vi "RSZVB Get Source Power Calibration Port State.vi"(8 "error in (no error)":errorcluster {"code" format="%.0x"}, 9 "Port Number (1)":i32=1, 10 "Channel (1)":i32=1, 11 "VISA session":refnum<visa-resource-name>) -> (0 "error out":errorcluster {"code" format="%.0x"}, 2 "Port State":bool, 3 "dup VISA session":refnum<visa-resource-name>)   [LabVIEW 2011]
doc: "This VI returns the state of the source power calibration for channel <Ch> and for port number <Pt>. \n\nNotes:\n\n(1) The command is disabled unless a source power calibration for the analyzer port has been performed (rszvb_InitiateSourcePowerCalibration). \n\n(2) To enable or disable a source power calibration for an external generator use SOURce<Ch>:POWer<Pt>:CORRection:GENerator[:STATe].\n\nRemote-control command(s):\nSOURce<Ch>:POWer<Pt>:CORRection[:STATe]?"
uses:
  _utility/RSZVB Global Data.vi
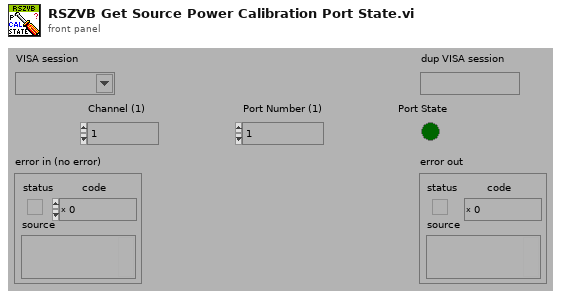
[diagram p1: front panel]
types:
  T1 = cluster{"Error Checking (T: On)":bool, "Installed Options":string[], "Data Valid?":bool, "Ports":i32, "Model":string[], "Option Checking (T: On)":bool}[]
  T2 = cluster{"Error Checking (T: On)":bool, "Installed Options":string[], "Data Valid?":bool, "Ports":i32, "Model":string[], "Option Checking (T: On)":bool}
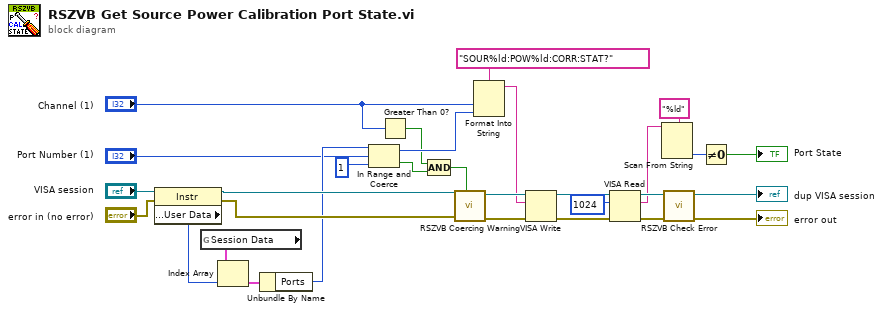
[diagram p0: block diagram]
diagram:
  n1 = property class="Instr"(reference="VISA session", error in="error in (no error)") -> (reference out=w12:refnum<visa-resource-name>, error out=w11:errorcluster, "General Settings:User Data"=w16:u32)
  n2 = global read "RSZVB Global Data.vi" "Session Data"() -> (w17:T1)
  n3 = Index Array(array=w17, index=w16) -> (element=w18:T2)
  n4 = Unbundle By Name(w18) -> ("Ports"=w8:i32)
  n5 = In Range and Coerce(upper limit=w8, x="Port Number (1)", lower limit=1) -> (coerced(x)=w6:i32, In Range?=w9:bool)
  n6 = Greater Than 0?(x="Channel (1)") -> (x > 0?=w2:bool)
  n7 = Compound Arithmetic op=AND(w2, w9) -> (w1:bool)
  n8 = call "RSZVB Coercing Warning.vi"("In Range?"=w1, "error in (no error)"=w11, "VISA session"=w12) -> ("error out"=w28:errorcluster, "dup VISA session"=w29:refnum<visa-resource-name>)  [unwired: 7 in]
  n9 = Format Into String(format string="SOUR%ld:POW%ld:CORR:STAT?", "Channel (1)", w6) -> (resulting string=w27:string)  [unwired: 2 in, 1 out]
  n10 = VISA Write(VISA resource name=w29, write buffer=w27, error in (no error)=w28) -> (VISA resource name out=w20:refnum<visa-resource-name>, error out=w19:errorcluster)  [unwired: 1 out]
  n11 = VISA Read(VISA resource name=w20, byte count=u32 1024 ("byte count (0)"), error in (no error)=w19) -> (VISA resource name out=w25:refnum<visa-resource-name>, read buffer=w22:string, error out=w24:errorcluster)  [unwired: 1 out]
  n12 = Scan From String(format string="%ld", input string=w22) -> (output 1=w21:i32)  [unwired: 3 in, 3 out]
  n13 = call "RSZVB Check Error.vi"("error in (no error)"=w24, "VISA session"=w25) -> ("error out"=→"error out":errorcluster, "dup VISA session"=→"dup VISA session":refnum<visa-resource-name>)  [unwired: 8 in]
  n14 = Not Equal To 0?(x=w21) -> (x != 0?=→"Port State":bool)
